vi "Zernike to Data.vi"(8 "error in (no error)":errorcluster, 11 "Zernike modes in":dbl[](array[slide]) scale=-1.0..1.0) -> (0 "error out":errorcluster, 2 "2D Data Out":dbl[][](array[numeric]), 3 "1D Data Out":dbl[](array[numeric]))   [LabVIEW 2015, in "DM.lvlib"]
uses:
  DM.lvlib
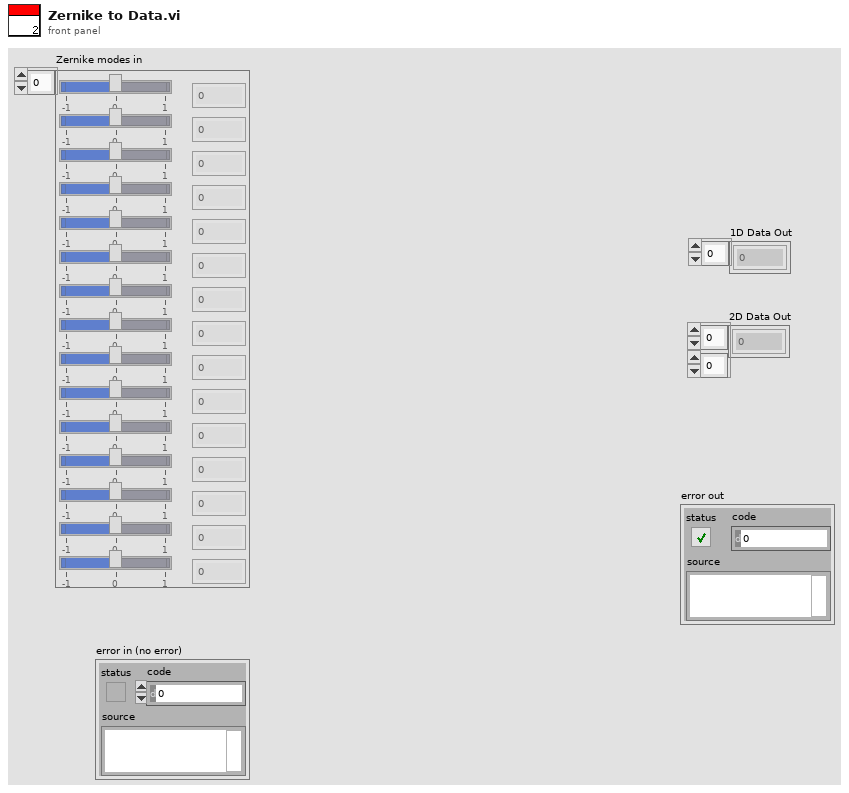
[diagram p1: front panel]
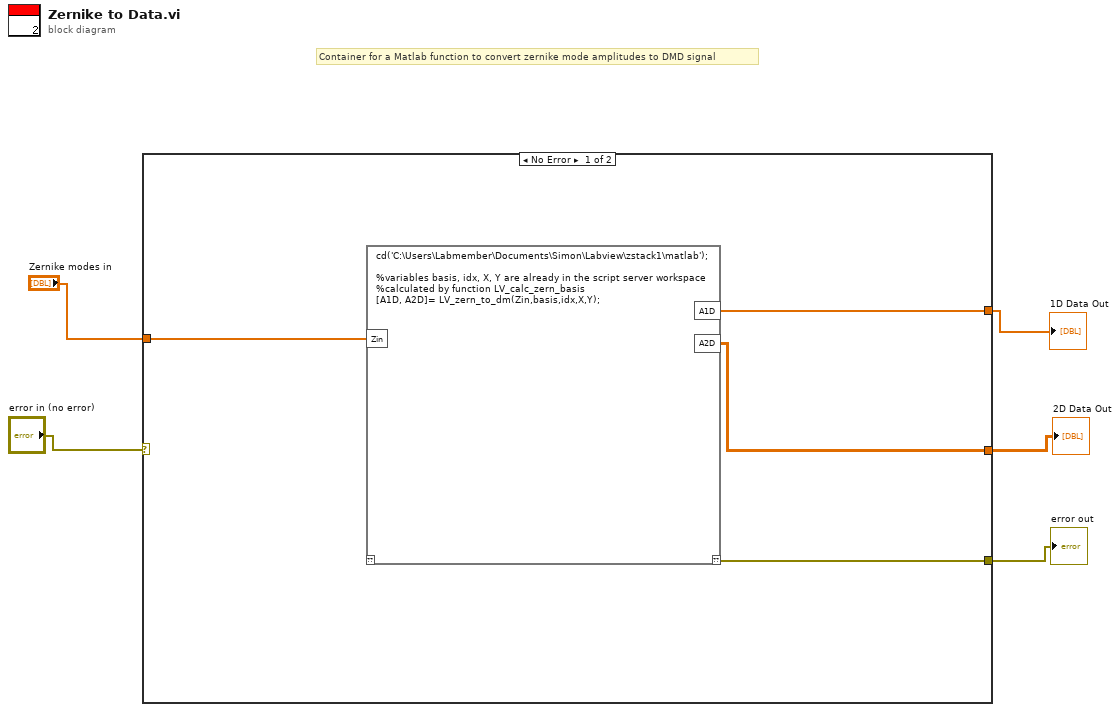
[diagram p0: block diagram]
diagram:
  # "Container for a Matlab function to convert zernike mode amplitudes to DMD signal"
  n1 = case shown="No Error" "error in (no error)" {
    selector: "error in (no error)" -> [_ w10]
    tunnel: "Zernike modes in" -> [w9 _]
    tunnel: [w8 _] -> w3
    tunnel: [w7 _] -> w2
    tunnel: [w6 w10] -> w1
    frame No Error {
      n2 = script code="cd('C:\\Users\\Labmember\\Documents\\Simon\\Labview\\zstack1\\matlab');\n\n%variables basis, idx, X, Y are already in the script server workspace\n%calculated by function LV_calc_zern_basis\n[A1D, A2D]= LV_zern_to_dm(Zin,basis,idx,X,Y);"("Zin"=w9) -> ("??"=w6:errorcluster, "A1D"=w8:dbl[], "A2D"=w7:dbl[][])  [unwired: 1 in]
    }
    frame Error {
    }
  }
  "2D Data Out" <- w2
  "1D Data Out" <- w3
  "error out" <- w1
